vi "TCP Loop.vi"(8 "error in":errorcluster, 10 "Queues":T1, 11 "Notifiers":T2) -> (0 "error out":errorcluster)   [LabVIEW 2014, in "TCP.lvlib"]
uses:
  TCP.lvlib
  support/Message Queue/Message Queue.lvlib
  <vilib>/ErrorRing/Error Ring.xnode
  TypeDefs/TCP Data.ctl
  Model/Model.lvlib
  PLC/PLC.lvlib
  <vilib>/Utility/error.llb/Error Cluster From Error Code.vi
  Support/Global names.vi
  SubVIs/TCP global names.vi
  Support/Message Queue/Message Cluster.ctl
  Support/Notifiers/Notifiers.ctl
  Support/Notifiers/Notifiers.lvlib
  Support/Message Queue/All Message Queues.ctl
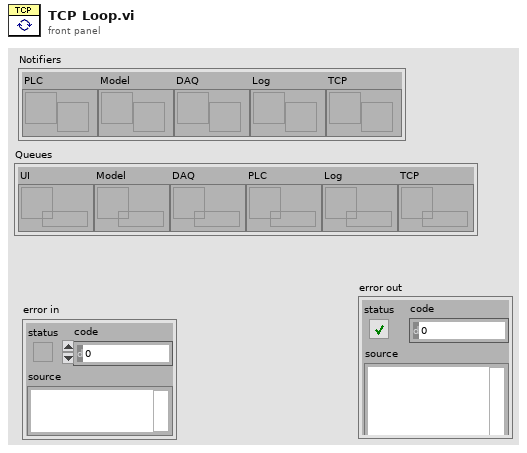
[diagram p1: front panel]
types:
  T1 = typedef "Message Queue.lvlib/All Message Queues.ctl" = cluster{"UI":refnum<queue>, "Model":refnum<queue>, "DAQ":refnum<queue>, "PLC":refnum<queue>, "Log":refnum<queue>, "TCP":refnum<queue>}
  T2 = typedef "Notifiers.lvlib/Notifiers.ctl" = cluster{"PLC":refnum<notifier>, "Model":refnum<notifier>, "DAQ":refnum<notifier>, "Log":refnum<notifier>, "TCP":refnum<notifier>}
  T3 = typedef "TCP.lvlib/TCP Data.ctl" = cluster{"Type":enum16{"Server", "Client"}, "IP":string, "Port":u16, "connection ID":refnum<k5>, "Connected?":bool, "Data":string}
  T4 = enum16{"Standard", "Buffered", "CRLF", "Immediate"}
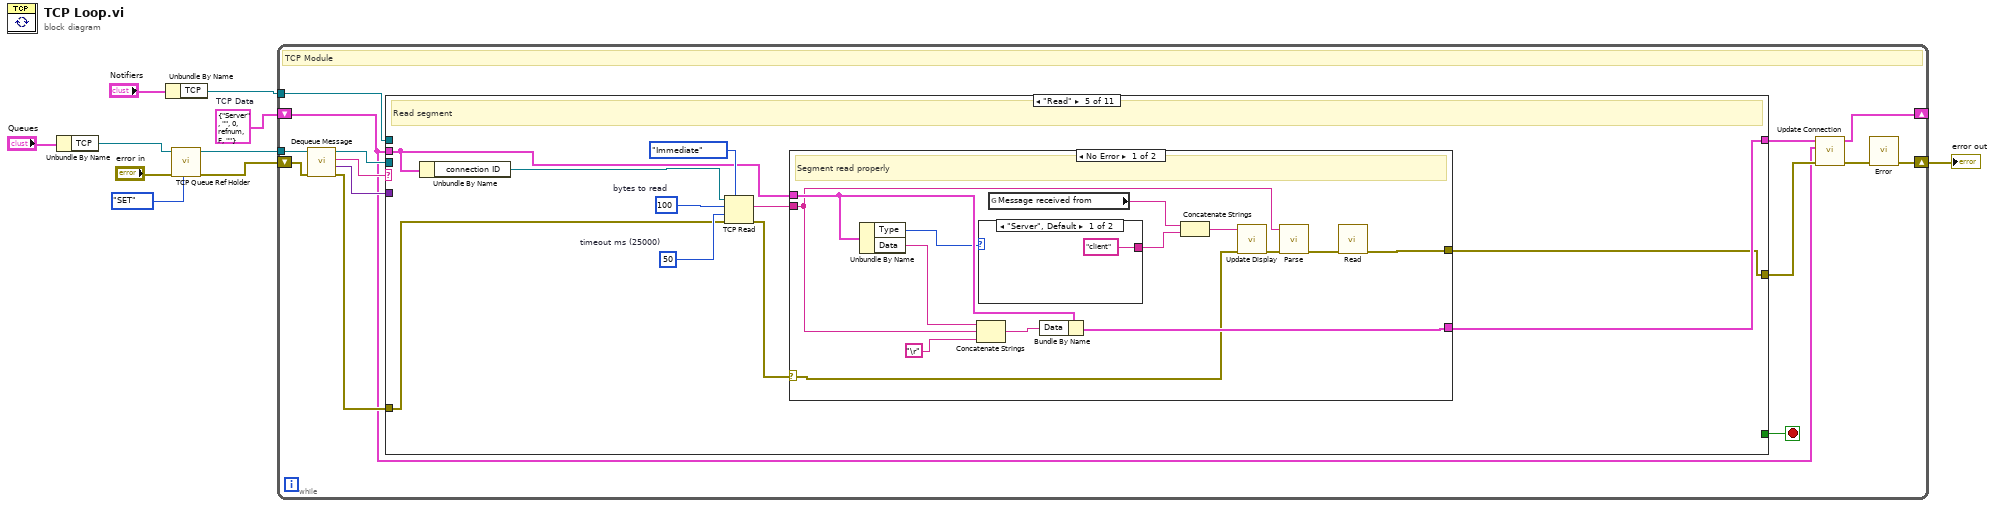
[diagram p0: block diagram]
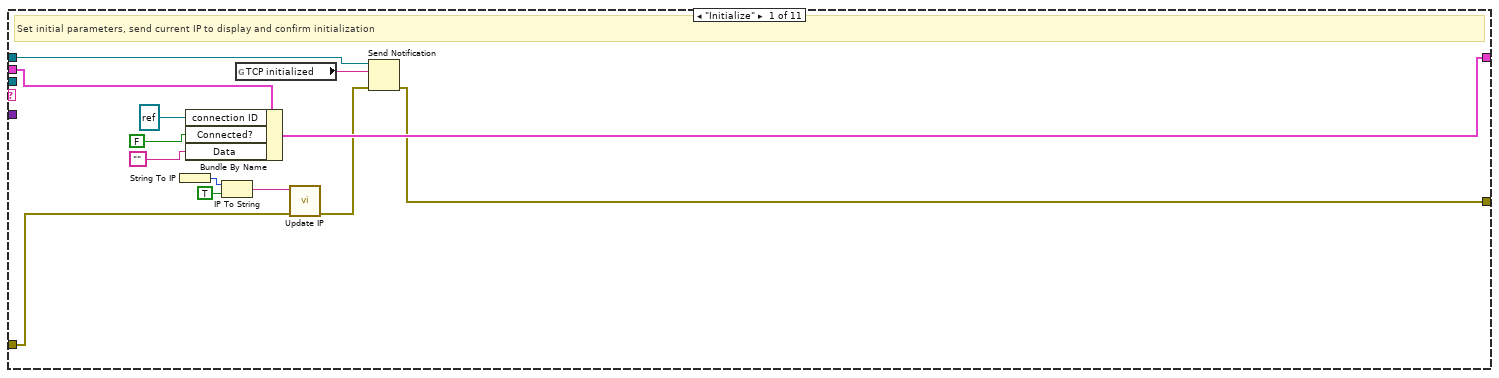
[diagram p2: hidden frame]
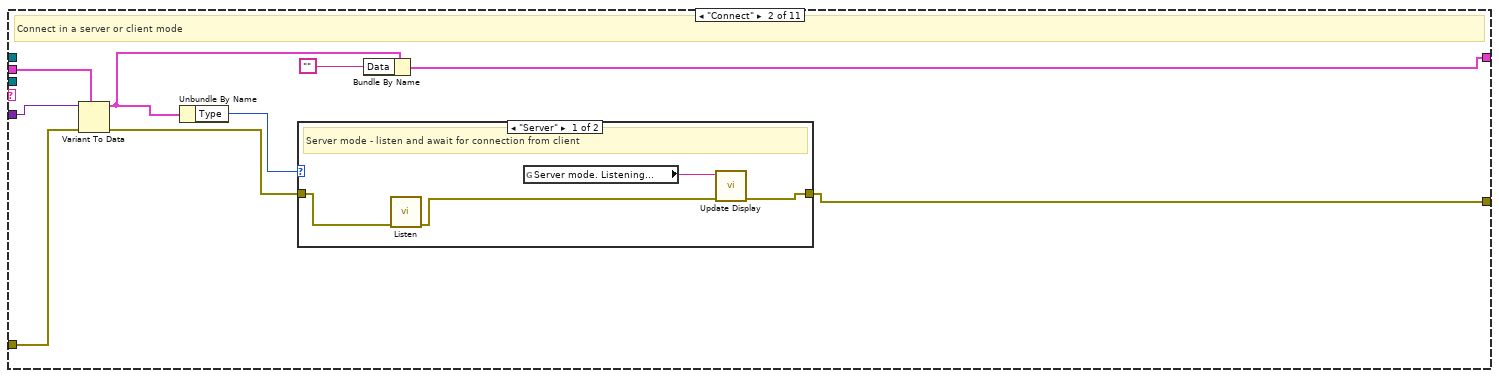
[diagram p3: hidden frame]
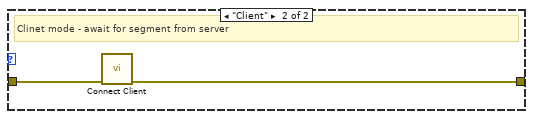
[diagram p4: hidden frame]
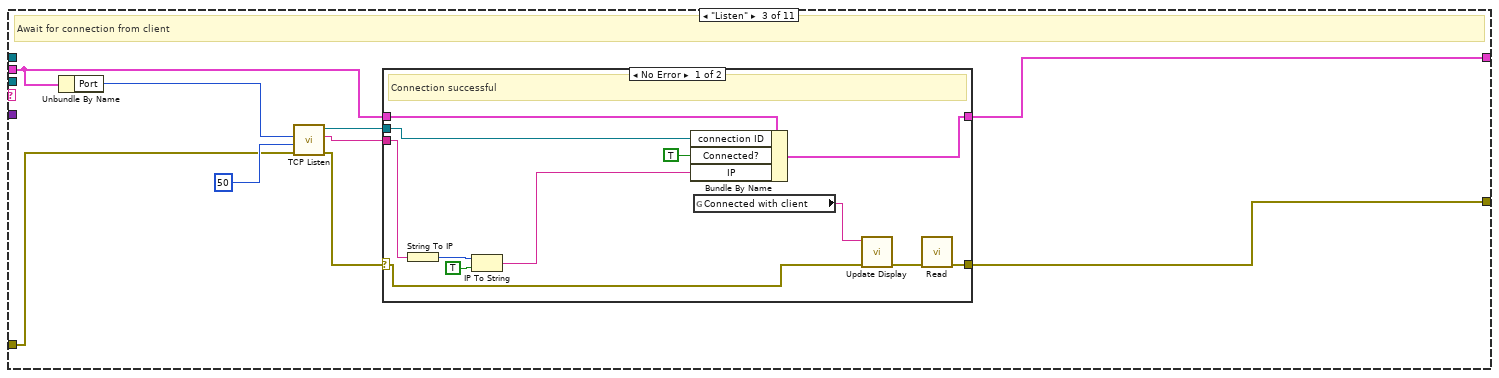
[diagram p5: hidden frame]
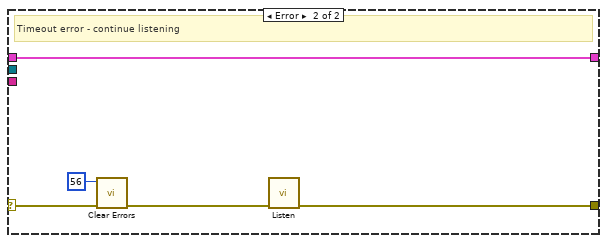
[diagram p6: hidden frame]
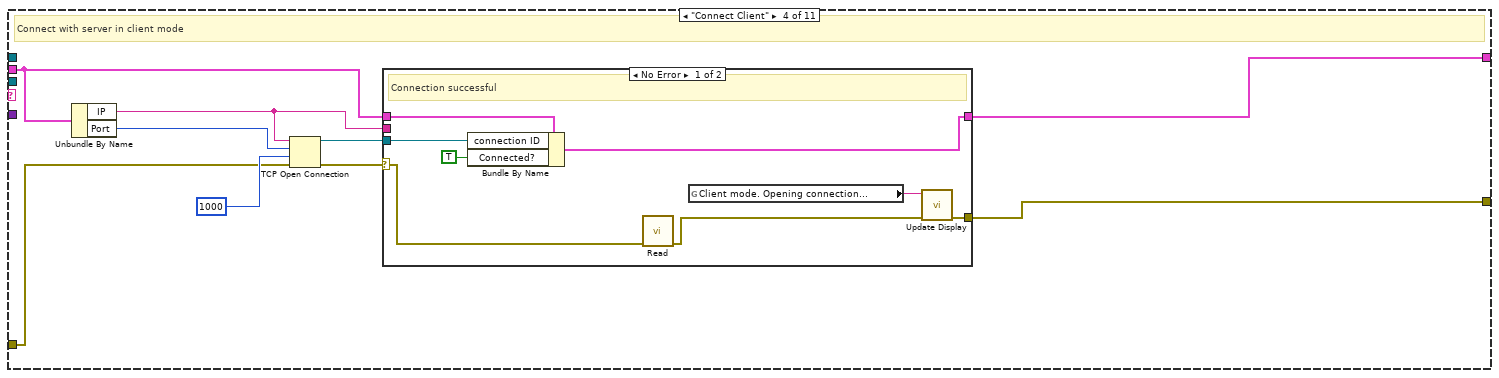
[diagram p7: hidden frame]
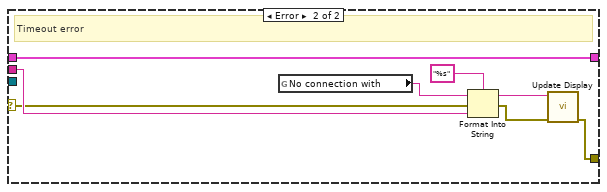
[diagram p8: hidden frame]
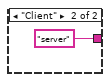
[diagram p9: hidden frame]
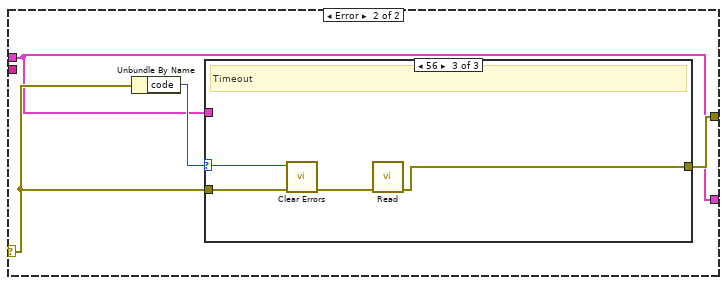
[diagram p10: hidden frame]
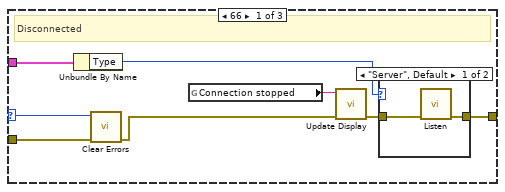
[diagram p11: hidden frame]
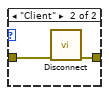
[diagram p12: hidden frame]
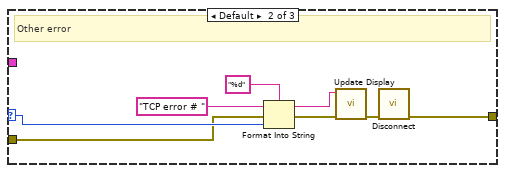
[diagram p13: hidden frame]
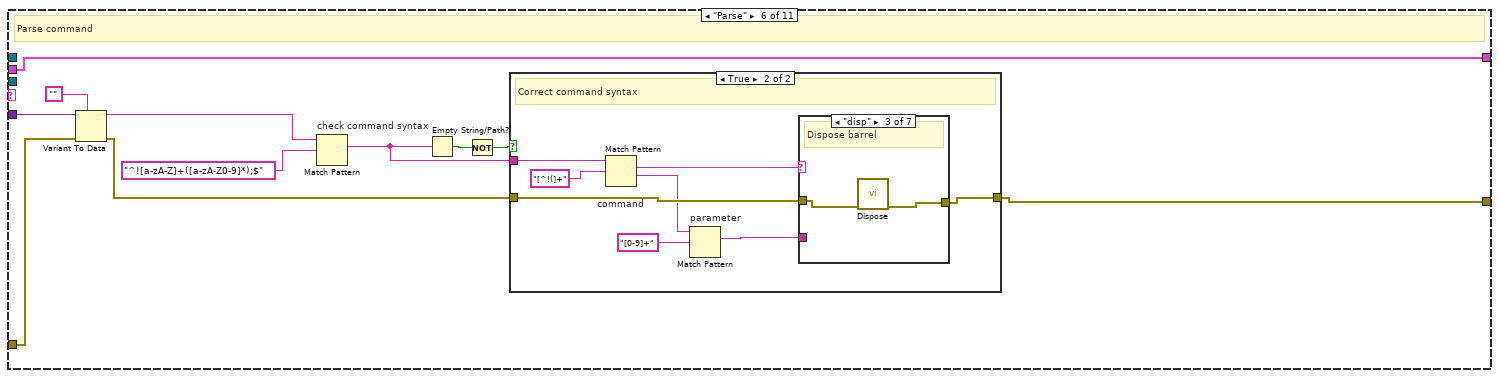
[diagram p14: hidden frame]
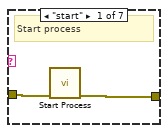
[diagram p16: hidden frame]
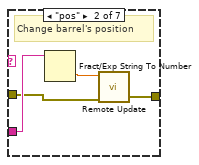
[diagram p17: hidden frame]
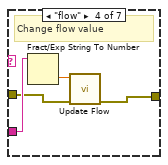
[diagram p18: hidden frame]
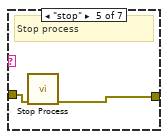
[diagram p19: hidden frame]
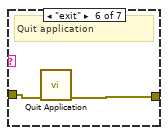
[diagram p20: hidden frame]
diagram:
  w10 = T3 {"Type"=enum."Server", "IP"="", "Port"=0, "connection ID"=refnum, "Connected?"=FALSE, "Data"=""}  # TCP Data
  n1 = Unbundle By Name("Queues") -> ("TCP"=w3:refnum<queue>)
  n2 = Unbundle By Name("Notifiers") -> ("TCP"=w4:refnum<notifier>)
  n3 = call "TCP Queue Ref Holder.vi"("Action"=enum16{"GET", "SET"}."SET", "error in"="error in", "Message Queue In"=w3) -> ("error out"=w7:errorcluster, "Input Message Queue"=w9:refnum<queue>)  [unwired: 7 in]
  n4 = while {
    tunnel: w9 -> [w24]
    tunnel: w4 -> [w19]
    shift-right: [w14] -> _
    shift-left: w10 -> [w11]
    shift-right: [w13] -> w1
    shift-left: w7 -> [w23]
    stop <- w20 stop-if-true
    # "TCP Module"
    n5 = call "Dequeue Message.vi"("error in (no error)"=w23, "Message Queue"=w24) -> ("error out"=w21:errorcluster, "Message Data"=w18:variant, "Message"=w22:string, "dup Message Queue"=w12:refnum<queue>)  [unwired: 6 in]
    n6 = case shown="\"Read\"" w22 {
      selector: w22 -> [_ _ _ _ _ _ _ _ _ _ w258]
      tunnel: w21 -> [w28 w46 w54 w79 w104 w166 w202 w228 w237 w255 _]
      tunnel: [w30 w45 w58 w82 w105 w163 w196 w224 w238 w252 w257] -> w17
      tunnel: [_ _ _ _ _ _ _ _ _ TRUE _] -> w20
      tunnel: w19 -> [w29 _ _ _ _ _ _ _ _ w250 _]
      tunnel: w11 -> [w37 w39 w56 w84 w107 w165 w199 w232 w236 w248 w256]
      tunnel: [w36 w43 w55 w83 w106 w165 w200 w233 w236 w247 w256] -> w15
      tunnel: w18 -> [_ w44 _ _ _ w168 w201 _ _ _ _]
      tunnel: w12 -> [_ _ _ _ _ _ _ w223 _ w245 _]
      frame "Initialize" {
        # "Set initial parameters, send current IP to display and confirm initialization"
        n7 = String To IP() -> (0:w31:u32)  [unwired: 1 in]
        n8 = Bundle By Name(cluster=w37, "connection ID"=refnum<k5> refnum, "Connected?"=FALSE, "Data"="") -> (w36:T3)
        n9 = IP To String(1:TRUE ("dot notation? (F)"), 2:w31) -> (0:w25:string)
        n10 = global read "Global names.vi" "TCP initialized"() -> (w26:string)
        n11 = call "Update IP.vi"("error in"=w28, "Message string"=w25) -> ("error out"=w27:errorcluster)  [unwired: 9 in]
        n12 = Send Notification(notification=w26, notifier=w29, error in (no error)=w27) -> (error out=w30:errorcluster)  [unwired: 1 out]
      }
      frame "Connect" {
        # "Connect in a server or client mode"
        n13 = Variant To Data(error in=w46, type=w39, Variant=w44) -> (data=w38:T3, error out=w42:errorcluster)
        n14 = Unbundle By Name(w38) -> ("Type"=w40:enum16{"Server", "Client"})
        n15 = case shown="\"Server\"" w40 {
          tunnel: w42 -> [w50 w52]
          tunnel: [w48 w51] -> w45
          frame "Server" {
            # "Server mode - listen and await for connection from client"
            n16 = call "Listen.vi"("error in"=w50) -> ("error out"=w49:errorcluster)  [unwired: 10 in]
            n17 = global read "TCP global names.vi" "Server mode. Listening..."() -> (w47:string)
            n18 = call "Update Display.vi"("error in"=w49, "Message string"=w47) -> ("error out"=w48:errorcluster)  [unwired: 9 in]
          }
          frame "Client" {
            # "Clinet mode - await for segment from server"
            n19 = call "Connect Client.vi"("error in"=w52) -> ("error out"=w51:errorcluster)  [unwired: 10 in]
          }
        }
        n20 = Bundle By Name(cluster=w38, "Data"="") -> (w43:T3)
      }
      frame "Listen" {
        # "Await for connection from client"
        n21 = Unbundle By Name(w56) -> ("Port"=w61:u16)
        n22 = call <vilib>:"TCP Listen.vi"("error in (no error)"=w54, "timeout ms (wait forever: -1)"=50, "port"=w61) -> ("error out"=w59:errorcluster, "remote address"=w53:string, "connection ID"=w57:refnum<k5>)  [unwired: 4 in, 2 out]
        n23 = case shown="No Error" w59 {
          selector: w59 -> [w62 w74]
          tunnel: [w68 w76] -> w58
          tunnel: w57 -> [w72 _]
          tunnel: w56 -> [w73 w77]
          tunnel: [w70 w77] -> w55
          tunnel: w53 -> [w66 _]
          frame No Error {
            # "Connection successful"
            n24 = String To IP(1:w66) -> (0:w65:u32)
            n25 = IP To String(1:TRUE ("dot notation? (F)"), 2:w65) -> (0:w63:string)
            n26 = Bundle By Name(cluster=w73, "connection ID"=w72, "Connected?"=TRUE, "IP"=w63) -> (w70:T3)
            n27 = global read "TCP global names.vi" "Connected with client"() -> (w67:string)
            n28 = call "Update Display.vi"("error in"=w62, "Message string"=w67) -> ("error out"=w69:errorcluster)  [unwired: 9 in]
            n29 = call "Read.vi"("error in"=w69) -> ("error out"=w68:errorcluster)  [unwired: 10 in]
          }
          frame Error {
            # "Timeout error - continue listening"
            n30 = call <vilib>:"Clear Errors.vi"("error in (no error)"=w74, "specific error code to clear (0: all)"=56) -> ("error out"=w75:errorcluster)  [unwired: 4 in, 1 out]
            n31 = call "Listen.vi"("error in"=w75) -> ("error out"=w76:errorcluster)  [unwired: 10 in]
          }
        }
      }
      frame "Connect Client" {
        # "Connect with server in client mode"
        n32 = Unbundle By Name(w84) -> ("IP"=w81:string, "Port"=w80:u16)
        n33 = TCP Open Connection(address=w81, remote port or service name=w80, timeout ms (60000)=1000, error in (no error)=w79) -> (connection ID=w85:refnum<k5>, error out=w86:errorcluster)  [unwired: 1 in]
        n34 = case shown="No Error" w86 {
          selector: w86 -> [w89 w98]
          tunnel: [w92 w97] -> w83
          tunnel: w85 -> [w94 _]
          tunnel: w84 -> [w95 w97]
          tunnel: [w91 w100] -> w82
          tunnel: w81 -> [_ w102]
          frame No Error {
            # "Connection successful"
            n35 = Bundle By Name(cluster=w95, "connection ID"=w94, "Connected?"=TRUE) -> (w92:T3)
            n36 = call "Read.vi"("error in"=w89) -> ("error out"=w90:errorcluster)  [unwired: 10 in]
            n37 = global read "TCP global names.vi" "Client mode. Opening connection..."() -> (w88:string)
            n38 = call "Update Display.vi"("error in"=w90, "Message string"=w88) -> ("error out"=w91:errorcluster)  [unwired: 9 in]
          }
          frame Error {
            # "Timeout error"
            n39 = global read "TCP global names.vi" "No connection with"() -> (w96:string)
            n40 = Format Into String(format string="%s", initial string=w96, error in=w98, w102) -> (resulting string=w99:string, error out=w101:errorcluster)
            n41 = call "Update Display.vi"("error in"=w101, "Message string"=w99) -> ("error out"=w100:errorcluster)  [unwired: 9 in]
          }
        }
      }
      frame "Read" {
        w111 = 50  # timeout ms (25000)
        w112 = 100  # bytes to read
        # "Read segment"
        n42 = Unbundle By Name(w107) -> ("connection ID"=w113:refnum<k5>)
        n43 = TCP Read(connection ID=w113, bytes to read=w112, error in (no error)=w104, 7:T4."Immediate" ("mode (standard)"), 9:w111) -> (data out=w108:string, error out=w109:errorcluster)  [unwired: 1 out]
        n44 = case shown="No Error" w109 {
          selector: w109 -> [w117 w132]
          tunnel: [w127 w130] -> w106
          tunnel: w108 -> [w121 _]
          tunnel: w107 -> [w126 w130]
          tunnel: [w118 w131] -> w105
          frame No Error {
            # "Segment read properly"
            n45 = Unbundle By Name(w126) -> ("Type"=w124:enum16{"Server", "Client"}, "Data"=w115:string)
            n46 = Concatenate Strings(w115, w121, "\r") -> (w125:string)
            n47 = case shown="\"Server\", Default" w124 {
              tunnel: ["client" ("Message") "server" ("f")] -> w123
              frame "Server", Default {
              }
              frame "Client" {
              }
            }
            n48 = global read "TCP global names.vi" "Message received from"() -> (w116:string)
            n49 = Bundle By Name(cluster=w126, "Data"=w125) -> (w127:T3)
            n50 = Concatenate Strings(w116, w123) -> (w120:string)
            n51 = call "Update Display.vi"("error in"=w117, "Message string"=w120) -> ("error out"=w122:errorcluster)  [unwired: 9 in]
            n52 = call "Parse.vi"("error in"=w122, "String"=w121) -> ("error out"=w119:errorcluster)  [unwired: 9 in]
            n53 = call "Read.vi"("error in"=w119) -> ("error out"=w118:errorcluster)  [unwired: 10 in]
          }
          frame Error {
            n54 = Unbundle By Name(w132) -> ("code"=w133:i32)
            n55 = case shown="56" w133 {
              selector: w133 -> [w134 w151 w154]
              tunnel: w132 -> [w137 w146 w155]
              tunnel: w130 -> [w141 _ _]
              tunnel: [w135 w147 w156] -> w131
              frame 66 {
                # "Disconnected"
                n56 = Unbundle By Name(w141) -> ("Type"=w140:enum16{"Server", "Client"})
                n57 = call <vilib>:"Clear Errors.vi"("error in (no error)"=w137, "specific error code to clear (0: all)"=w134) -> ("error out"=w136:errorcluster)  [unwired: 4 in, 1 out]
                n58 = global read "TCP global names.vi" "Connection stopped"() -> (w139:string)
                n59 = call "Update Display.vi"("error in"=w136, "Message string"=w139) -> ("error out"=w138:errorcluster)  [unwired: 9 in]
                n60 = case shown="\"Server\", Default" w140 {
                  tunnel: w138 -> [w142 w144]
                  tunnel: [w143 w145] -> w135
                  frame "Server", Default {
                    n61 = call "Listen.vi"("error in"=w142) -> ("error out"=w143:errorcluster)  [unwired: 10 in]
                  }
                  frame "Client" {
                    n62 = call "Disconnect.vi"("error in"=w144) -> ("error out"=w145:errorcluster)  [unwired: 10 in]
                  }
                }
              }
              frame Default {
                # "Other error"
                n63 = Format Into String(format string="%d", initial string="TCP error # " ("Message"), error in=w146, w151) -> (resulting string=w149:string, error out=w150:errorcluster)
                n64 = call "Update Display.vi"("error in"=w150, "Message string"=w149) -> ("error out"=w148:errorcluster)  [unwired: 9 in]
                n65 = call "Disconnect.vi"("error in"=w148) -> ("error out"=w147:errorcluster)  [unwired: 10 in]
              }
              frame 56 {
                # "Timeout"
                n66 = call <vilib>:"Clear Errors.vi"("error in (no error)"=w155, "specific error code to clear (0: all)"=w154) -> ("error out"=w157:errorcluster)  [unwired: 4 in, 1 out]
                n67 = call "Read.vi"("error in"=w157) -> ("error out"=w156:errorcluster)  [unwired: 10 in]
              }
            }
          }
        }
      }
      frame "Parse" {
        # "Parse command"
        n68 = Variant To Data(error in=w166, type="", Variant=w168) -> (data=w159:string, error out=w164:errorcluster)
        n69 = Match Pattern "check command syntax"(string=w159, regular expression="^![a-zA-Z]+([a-zA-Z0-9]*);$") -> (match substring=w162:string)  [unwired: 1 in, 3 out]
        n70 = Empty String/Path?(string/path=w162) -> (empty?=w161:bool)
        n71 = Not(x=w161) -> (.not. x?=w160:bool)
        n72 = case shown="True" w160 {
          tunnel: w162 -> [_ w177]
          tunnel: w164 -> [w169 w175]
          tunnel: [w169 w173] -> w163
          frame False {
            # "Incorrect command"
          }
          frame True {
            # "Correct command syntax"
            n73 = Match Pattern "command"(string=w177, regular expression="[^!(]+" ("remove start/stop signs")) -> (match substring=w172:string, after substring=w171:string)  [unwired: 1 in, 2 out]
            n74 = Match Pattern "parameter"(string=w171, regular expression="[0-9]+" ("parameter")) -> (match substring=w170:string)  [unwired: 1 in, 3 out]
            n75 = case shown="\"disp\"" w172 {
              tunnel: w175 -> [w179 w180 w185 w186 w191 w193 w194]
              tunnel: [w178 w183 w184 w189 w190 w192 w194] -> w173
              tunnel: w170 -> [_ w182 _ w188 _ _ _]
              frame "start" {
                # "Start process"
                n76 = call "Start Process.vi"("error in"=w179) -> ("error out"=w178:errorcluster)  [unwired: 10 in]
              }
              frame "pos" {
                # "Change barrel's position"
                n77 = Fract/Exp String To Number(string=w182) -> (number=w181:dbl)  [unwired: 3 in, 1 out]
                n78 = call "Remote Update.vi"("error in"=w180, "Value"=w181) -> ("error out"=w183:errorcluster)  [unwired: 9 in]
              }
              frame "disp" {
                # "Dispose barrel"
                n79 = call "Dispose.vi"("error in (no error)"=w185) -> ("error out"=w184:errorcluster)  [unwired: 10 in]
              }
              frame "flow" {
                # "Change flow value"
                n80 = Fract/Exp String To Number(string=w188) -> (number=w187:dbl)  [unwired: 3 in, 1 out]
                n81 = call "Update Flow.vi"("error in (no error)"=w186, "Flow"=w187) -> ("error out"=w189:errorcluster)  [unwired: 9 in]
              }
              frame "stop" {
                # "Stop process"
                n82 = call "Stop Process.vi"("error in"=w191) -> ("error out"=w190:errorcluster)  [unwired: 10 in]
              }
              frame "exit" {
                # "Quit application"
                n83 = call "Quit Application.vi"("error in"=w193) -> ("error out"=w192:errorcluster)  [unwired: 10 in]
              }
              frame Default {
                # "Improper parameters"
              }
            }
          }
        }
      }
      frame "Send" {
        # "Send segment"
        n84 = Unbundle By Name(w199) -> ("Connected?"=w198:bool)
        n85 = case shown="True" w198 {
          tunnel: w202 -> [w205 w220]
          tunnel: w201 -> [_ w219]
          tunnel: w199 -> [w204 w209]
          tunnel: [w204 w209] -> w200
          tunnel: [w203 w212] -> w195
          tunnel: [w205 w210] -> w197
          frame False {
            n86 = global read "TCP global names.vi" "No connection - data not sent!"() -> (w203:string)
          }
          frame True {
            w215 = 1000  # timeout
            n87 = Variant To Data(error in=w220, type="", Variant=w219) -> (data=w206:string, error out=w211:errorcluster)
            n88 = Unbundle By Name(w209) -> ("Type"=w214:enum16{"Server", "Client"}, "connection ID"=w207:refnum<k5>)
            n89 = case shown="\"Server\", Default" w214 {
              tunnel: ["client" ("Message") "server" ("f")] -> w213
              frame "Server", Default {
              }
              frame "Client" {
              }
            }
            n90 = TCP Write(connection ID=w207, data in=w206, error in (no error)=w211, 9:w215) -> (error out=w217:errorcluster)  [unwired: 2 out]
            n91 = global read "TCP global names.vi" "Message sent to"() -> (w208:string)
            n92 = call <vilib>:"Clear Errors.vi"("error in (no error)"=w217, "specific error code to clear (0: all)"=56) -> ("error out"=w210:errorcluster)  [unwired: 4 in, 1 out]
            n93 = Concatenate Strings(w208, w213) -> (w212:string)
          }
        }
        n94 = call "Update Display.vi"("error in"=w197, "Message string"=w195) -> ("error out"=w196:errorcluster)  [unwired: 9 in]
      }
      frame "Disconnect" {
        # "Disconnect"
        n95 = Unbundle By Name(w232) -> ("connection ID"=w231:refnum<k5>)
        n96 = Flush Queue(queue=w223, error in (no error)=w228) -> (error out=w227:errorcluster)  [unwired: 2 out]
        n97 = TCP Close Connection(connection ID=w231, error in (no error)=w227) -> (error out=w226:errorcluster)  [unwired: 1 in, 1 out]
        n98 = Bundle By Name(cluster=w232, "Connected?"=FALSE) -> (w233:T3)
        n99 = call "Update Display.vi"("error in"=w226, "Message string"="Connection closed" ("Message")) -> ("error out"=w225:errorcluster)  [unwired: 9 in]
        n100 = call <vilib>:"Clear Errors.vi"("error in (no error)"=w225) -> ("error out"=w224:errorcluster)  [unwired: 5 in, 1 out]
      }
      frame "Say goodbye" {
        # "Send goodbye info"
        n101 = Unbundle By Name(w236) -> ("Connected?"=w234:bool, "IP"=w235:string)
        n102 = case shown="True" w234 {
          tunnel: [w239 w244] -> w238
          tunnel: w237 -> [w239 w243]
          tunnel: w235 -> [_ w242]
          frame False {
          }
          frame True {
            n103 = global read "TCP global names.vi" "Disconnected with"() -> (w240:string)
            n104 = Concatenate Strings(w240, w242) -> (w241:string)
            n105 = call "Send.vi"("error in"=w243, "Data"=w241) -> ("error out"=w244:errorcluster)  [unwired: 9 in]
          }
        }
      }
      frame "Exit" {
        # "Release queue, send exit notification and quit TCP loop"
        n106 = Bundle By Name(cluster=w248, "Connected?"=FALSE) -> (w247:T3)
        n107 = Release Queue(queue=w245, force destroy? (F)=TRUE, error in (no error)=w255) -> (error out=w253:errorcluster)  [unwired: 2 out]
        n108 = global read "Global names.vi" "TCP exit"() -> (w246:string)
        n109 = Send Notification(notification=w246, notifier=w250, error in (no error)=w253) -> (error out=w252:errorcluster)  [unwired: 1 out]
      }
      frame Default {
        # "Incorrect message"
        n110 = xnode "Error Ring"("parameter 0"=w258) -> ("error out"=w257:errorcluster)
      }
    }
    n111 = call "Update Connection.vi"("error in (no error)"=w17, "TCP Data before update"=w11, "TCP Data after update"=w15) -> ("error out"=w16:errorcluster, "TCP Data after update out"=w14:T3)  [unwired: 7 in]
    n112 = call "Error.vi"("error in"=w16) -> ("error out"=w13:errorcluster)  [unwired: 10 in]
  }
  "error out" <- w1
